vi "HBcenterFinder2Fids.vi"(0 "Operation":enum16{"Manual", "Automatic"}(ring)=enum."Automatic", 1 "Zone":enum16{"ZoneA", "ZoneB", "ZoneC", "ZoneD"}(ring), 2 "Autofocus":T3={"Enable"=TRUE, "InitialStepSize"=0.05, "Tolerance"=0.02, "Abort"=FALSE} {"Tolerance" format="%#_13g"}, 5 "Component":enum16{"BP", "Si", "HB", "HBonBP", "Other"}(ring)=enum."HB", 9 "VisibilityInCamera":enum16{"JoyStick", "AllVisible"}(ring)=enum."AllVisible", 11 "error in (no error)":errorcluster, 12 "Position":enum16{"1", "2"}(ring), 13 "SaveImagesLog":bool=TRUE) -> (4 "Output XYZU":string, 6 "Image":T4(plugin-control), 8 "Image 2":T4[](array[plugin-control]) caption="AllImages", 15 "error out":errorcluster)   [LabVIEW 2021]
uses:
  <vilib>/userDefined/High Color/IMAQdx.ctl
  <vilib>/Analysis/coordinate.llb/2D Cartesian Coordinate Rotation (Scalar).vi
  <vilib>/Analysis/baseanly.llb/Mean (DBL).vi
  include/GlobalVariables.vi
  <vilib>/Analysis/NI_AALPro.lvlib
  <vilib>/Analysis/NI_AALBase.lvlib
  <vilib>/vision/driver/NI_Vision_Acquisition_Software.lvlib
panel:
  out "JoyStickStatus":bool
  in  "YoffsetMidFid":dbl=3.5005
  in  "XoffsetMidFid":dbl
  out "DistFids":dbl=50.0
  out "AllMatches":T1(array[cluster]) {"Bounding Box"."y" format="%.2f"; "Bounding Box"."x" format="%.2f"; "Score" format="%.2f"; "Scale" format="%.2f"; "Angle" format="%.2f"; "Position"."y" format="%.2f"; "Position"."x" format="%.2f"}
  in  "Camera":T2="cam1"
  out "OutputFile":string
  out "spreadsheet string 2":string
  out "spreadsheet string":string
  in  "ModuleName":string="T1"
  out "SyringeY":dbl format="%#_7g"
  out "SyringeX":dbl format="%#_7g"
  in  "CamToSyringeYoffset":dbl=126.651
  in  "CamToSyringeXoffset":dbl=167.702
  out "FileUsedForFiducials":string
  out "UsedCoordinates":string
  out "CameraGcode":string
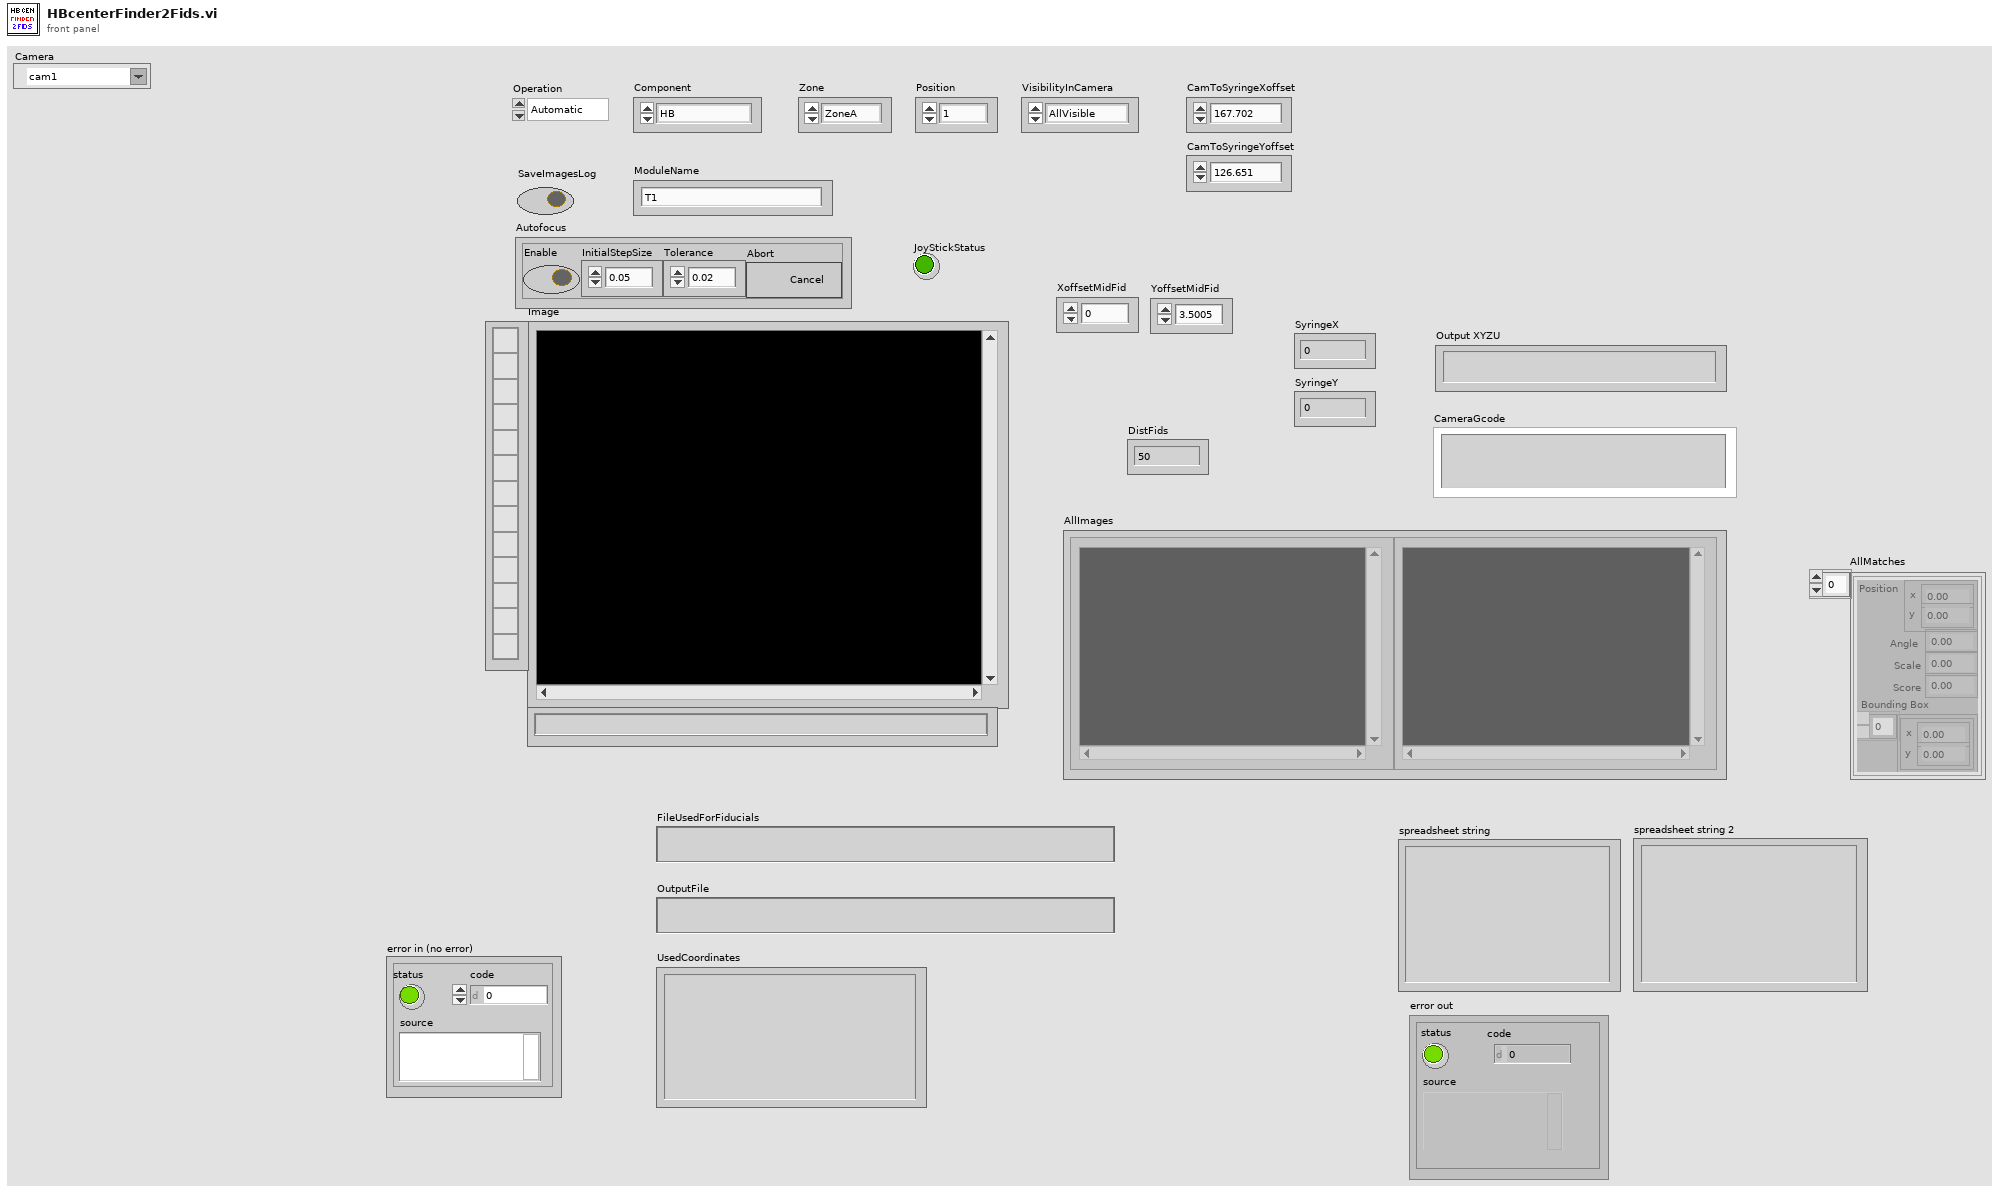
[diagram p1: front panel]
types:
  T1 = cluster{"Position":cluster{"x":sgl, "y":sgl}, "Angle":sgl, "Scale":sgl, "Score":sgl, "Bounding Box":cluster{"x":sgl, "y":sgl}[]}[]
  T2 = typedef "IMAQdx.ctl" = refnum<k21>
  T3 = cluster{"Enable":bool, "InitialStepSize":dbl, "Tolerance":dbl, "Abort":bool}
  T4 = typedef "IMAQ Image.ctl" = refnum<image>
  T5 = cluster{"Number of Matches Requested":i32, "Minimum Match Score":sgl, "Angle Ranges":cluster{"Start Angle":sgl, "End Angle":sgl}[]}
  T6 = typedef "Image Type" = u32
  T7 = typedef "IMAQ Circle" = cluster{"Center X":i32, "Center Y":i32, "Inner Radius":i32, "Outer Radius":i32, "Start Angle":dbl, "End Angle":dbl}
  T8 = enum16{"Left Button", "Center Button", "Right Button", "Window Close"}
  T9 = enum16{"open", "replace", "create", "open or create", "replace or create", "replace or create with confirmation"}
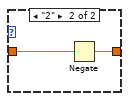
[diagram p2: hidden frame]
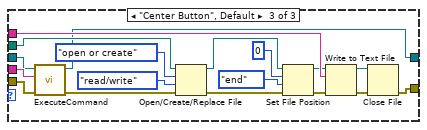
[diagram p5: hidden frame]
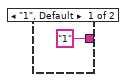
[diagram p6: hidden frame]
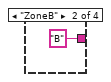
[diagram p7: hidden frame]
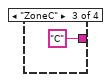
[diagram p8: hidden frame]
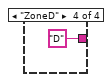
[diagram p9: hidden frame]
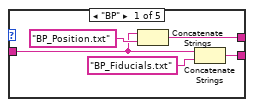
[diagram p10: hidden frame]
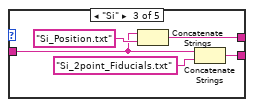
[diagram p11: hidden frame]
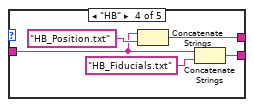
[diagram p12: hidden frame]
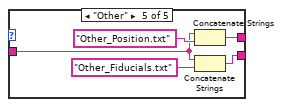
[diagram p13: hidden frame]
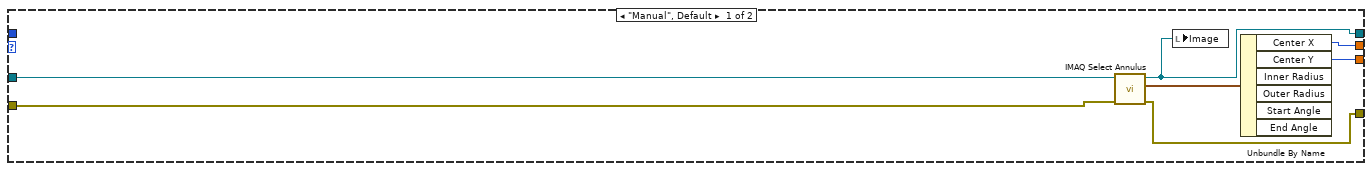
[diagram p14: hidden frame]
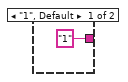
[diagram p16: hidden frame]
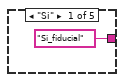
[diagram p17: hidden frame]
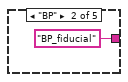
[diagram p18: hidden frame]
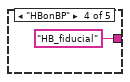
[diagram p19: hidden frame]
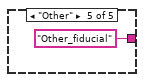
[diagram p20: hidden frame]
diagram:
  w49 = "%f" ("format string")
  w87 = "\t"
  w84 = i16 6 ("width (-)")
  # "Write the XYZU of the baseplate to a text file & move the gantry?"
  # "Prepare to move the gantry to see the center of baseplate in camera."
  # "AllVisble: Assumes that you know the coordinates of all corners (fiducials) well. No need for any adjustments.\nJoyStick: Use joystick at each point to make good image.\nClickMove: Use \"AdjustCamera\" panel and move the gantry stepwise. Click \"Done\" when you're satisfied with the picture."
  n1 = flat-sequence {
    tunnel: [w96] -> w45
    tunnel: w45 -> [w112]
    tunnel: [w111] -> w44
    tunnel: [w110] -> w42
    tunnel: [w109] -> w39
    tunnel: w44 -> [w164]
    tunnel: [w164] -> w43
    tunnel: w42 -> [w157]
    tunnel: [w152] -> w41
    tunnel: [w163] -> w40
    tunnel: w39 -> [w162]
    tunnel: [w162] -> w38
    tunnel: [w156] -> w30
    tunnel: [w155] -> w29
    tunnel: 2 -> [w191]
    tunnel: "VisibilityInCamera" -> [w184]
    tunnel: w43 -> [w182]
    tunnel: w41 -> [w174]
    tunnel: w40 -> [w181]
    tunnel: w38 -> [w180]
    tunnel: w30 -> [w172]
    tunnel: w29 -> [w173]
    tunnel: [w190] -> w28
    tunnel: [w189] -> w27
    tunnel: [w188] -> w26
    tunnel: [w187] -> w25
    tunnel: [w186] -> w24
    tunnel: [w185] -> w23
    tunnel: [w183] -> w22
    tunnel: [w180] -> w21
    tunnel: [w179] -> w20
    tunnel: [w171] -> w19
    tunnel: [w452] -> w36
    tunnel: [w453] -> w37
    tunnel: [w454] -> w54
    tunnel: [w455] -> w15
    tunnel: [w449] -> w16
    tunnel: [w456] -> _
    tunnel: [w457] -> w91
    tunnel: [w458] -> w50
    tunnel: [w459] -> w51
    tunnel: w28 -> [w459]
    tunnel: w27 -> [w458]
    tunnel: w26 -> [w457]
    tunnel: w25 -> [w456]
    tunnel: w24 -> [w450]
    tunnel: w23 -> [w455]
    tunnel: w22 -> [w454]
    tunnel: w21 -> [w453]
    tunnel: w20 -> [w452]
    tunnel: w19 -> [w451]
    frame #0 {
      n2 = case shown="\"ZoneA\", Default" "Zone" {
        tunnel: ["A" "B" "C" "D"] -> w100
        frame "ZoneA", Default {
        }
        frame "ZoneB" {
        }
        frame "ZoneC" {
        }
        frame "ZoneD" {
        }
      }
      n3 = case shown="\"2\"" "Position" {
        tunnel: ["1" "2"] -> w101
        frame "1", Default {
        }
        frame "2" {
        }
      }
      n4 = Concatenate Strings(w100, w101, "_" ("string")) -> (w96:string)
      "UsedCoordinates" <- ""
    }
    frame #1 {
      n5 = Concatenate Strings("C:\\Users\\TTUHEP\\Documents\\LabVIEW\\GantryPrograms\\", "Configs\\" ("string"), w112) -> (w119:string)
      n6 = case shown="\"HBonBP\"" "Component" {
        tunnel: w119 -> [w127 w132 w138 w143 w148]
        tunnel: [w128 w133 w140 w145 w150] -> w122
        tunnel: [w129 w134 w137 w142 w147] -> w109
        frame "BP" {
          n7 = Concatenate Strings(w127, "BP_Position.txt") -> (w129:string)
          n8 = Concatenate Strings(w127, "BP_Fiducials.txt") -> (w128:string)
        }
        frame "HBonBP" {
          n9 = Concatenate Strings(w132, "BP_Position.txt") -> (w134:string)
          n10 = Concatenate Strings(w132, "HBonBP_Fiducials.txt") -> (w133:string)
        }
        frame "Si" {
          n11 = Concatenate Strings(w138, "Si_Position.txt") -> (w137:string)
          n12 = Concatenate Strings(w138, "Si_2point_Fiducials.txt") -> (w140:string)
        }
        frame "HB" {
          n13 = Concatenate Strings(w143, "HB_Position.txt") -> (w142:string)
          n14 = Concatenate Strings(w143, "HB_Fiducials.txt") -> (w145:string)
        }
        frame "Other" {
          n15 = Concatenate Strings(w148, "Other_Position.txt") -> (w147:string)
          n16 = Concatenate Strings(w148, "Other_Fiducials.txt") -> (w150:string)
        }
      }
      "FileUsedForFiducials" <- w122
      "OutputFile" <- w109
      n17 = String To Path(string=w122) -> (path=w120:path)
      n18 = Concatenate Strings("This file does not exist:" ("ErrorMessage"), w122) -> (w123:string)
      n19 = call <vilib>:"Check if File or Folder Exists.vi"("error in (no error)"="error in (no error)", "path"=w120) -> ("error out"=w121:errorcluster, "file or folder exists?"=w124:bool, "dup path"=w111:path)  [unwired: 7 in]
      n20 = Not(x=w124) -> (.not. x?=w125:bool)
      n21 = call "AddError.vi"("NoErrorMessage"="InFile OK", "ErrorMessage"=w123, "error in"=w121, "code"=-995, "Error?"=w125) -> ("Error out"=w110:errorcluster)  [unwired: 6 in]
    }
    frame #2 {
      w158 = T6 0 items=["Grayscale (U8)", "Grayscale (I16)", "Grayscale (SGL)", "Complex (CSG)", "RGB (U32)", "HSL (U32)", "RGB (U64)", "Grayscale (U16)"] ("Image Type")
      # "Set the size of the window while selecting the point."
      n22 = call "IMAQ WindSize"("Scrollbars? (N)"=TRUE, "Width & Height"=cluster{"Width":i32, "Height":i32} {"Width"=1333, "Height"=1000}, "Window Number"=0) -> ()  [unwired: 3 in, 3 out]
      n23 = call "IMAQ Create"("Image Name"="name1" ("ImageName"), "Image Type"=w158, "error in (no error)"=w157) -> ("New Image"=w155:T4, "error out"=w160:errorcluster)  [unwired: 2 in]
      n24 = call "Connect.vi"("error in (no error)"=w157) -> ("error out"=w166:errorcluster, "controller"=w167:refnum<k24>)  [unwired: 9 in]
      n25 = call "ExecuteCommand.vi"("error in (no error)"=w166, "Command Code"="G90\nG1 Z0 F100", "controller in"=w167) -> ("error out"=w154:errorcluster, "controller out"=w163:refnum<k24>)  [unwired: 6 in, 1 out]
      n26 = call <vilib>:"IMAQdx Open Camera.vi"("error in"=w160, "Session In"="Camera") -> ("error out"=w153:errorcluster, "Session Out"=w156:T2)  [unwired: 8 in]
      n27 = Merge Errors(w154, w153) -> (w152:errorcluster)
    }
    frame #3 {
      n28 = local read "Autofocus"() -> (w176:T3)
      n29 = local read "Autofocus"() -> (w178:T3)
      n30 = Unbundle By Name(w178) -> ("Enable"=w177:bool)
      n31 = Unbundle By Name(w176) -> ("Abort"=w175:bool)
      n32 = for {
        N: w191 -> [_]
        tunnel: w181 -> [w252]
        tunnel: w182 -> [w235]
        tunnel: [w233] -> w190 mode=indexing
        tunnel: [w232] -> w189 mode=indexing
        tunnel: [w231] -> w188 mode=indexing
        tunnel: [w227] -> w187 mode=indexing
        tunnel: [w226] -> w185
        tunnel: w184 -> [w225]
        tunnel: w175 -> [w224]
        tunnel: w177 -> [w223]
        tunnel: [w219] -> w183
        tunnel: [w214] -> w179 mode=indexing
        shift-right: [w217] -> w186
        shift-left: w174 -> [w201]
        tunnel: w173 -> [w200]
        shift-right: [w194] -> w171
        shift-left: w172 -> [w193]
        i -> [w212]
        w203 = T6 6 items=["Grayscale (U8)", "Grayscale (I16)", "Grayscale (SGL)", "Complex (CSG)", "RGB (U32)", "HSL (U32)", "RGB (U64)", "Grayscale (U16)"] ("Image Type")
        # "Array of XY cluser"
        # "Z array"
        # "Y array"
        # "X array"
        # "Read text file line by line. Each line contains X,Y,Z coordinates for the gantry."
        n33 = call "GetArrayFmTxtFile.vi"("error in"=w201, "LineNo."=w212, "TextFile"=w235) -> ("error out"=w234:errorcluster, "Array"=w259:dbl[])
        n34 = Index Array(array=w259, index=0) -> (element=w254:dbl)
        n35 = Index Array(array=w259, index=1) -> (element=w253:dbl)
        n36 = Index Array(array=w259, index=2) -> (element=w255:dbl)
        n37 = call "Move.vi"("X"=w254, "Absolute"=TRUE, "Y"=w253, "Z"=w255, "SpeedXY (mm/s)"=100.0, "SpeedZ (mm/s)"=100.0, "Move Z first"=FALSE) -> ("Position Gcode"=w251:string)  [unwired: 8 in]
        n38 = call "ExecuteCommand.vi"("error in (no error)"=w234, "Command Code"=w251, "controller in"=w252) -> ("error out"=w199:errorcluster, "controller out"=w250:refnum<k24>)  [unwired: 6 in, 1 out]
        n39 = call <vilib>:"IMAQdx Snap2.vi"("error in"=w199, "Image In"=w200, "Session In"=w193) -> ("error out"=w198:errorcluster, "Image Out"=w196:T4, "Session Out"=w197:T2)  [unwired: 6 in]
        n40 = local write "Image"(w196) -> ()
        n41 = case shown="\"JoyStick\", Default" w225 {
          tunnel: w197 -> [w367 w418]
          tunnel: w250 -> [w384 w430]
          tunnel: w198 -> [w382 w431]
          tunnel: [w363 w419] -> w221
          tunnel: [w371 w425] -> w239
          tunnel: [w372 w423] -> w195
          tunnel: w224 -> [w375 w428]
          tunnel: w223 -> [w369 w429]
          tunnel: "name1" ("ImageName") -> [w368 w417]
          tunnel: w196 -> [w366 w416]
          tunnel: [w362 w415] -> w194
          frame "JoyStick", Default {
            # "Use joystick to go to a position where camera sees good image."
            n42 = while {
              tunnel: [w407] -> w364
              tunnel: w384 -> [w414]
              tunnel: [w412] -> w380
              tunnel: [w414] -> w381
              tunnel: w382 -> [w413]
              tunnel: w367 -> [w411]
              tunnel: w366 -> [w410]
              tunnel: [w409] -> w365
              stop <- w408 continue-if-true
              n43 = call <vilib>:"IMAQdx Snap2.vi"("error in"=w413, "Image In"=w410, "Session In"=w411) -> ("error out"=w412:errorcluster, "Image Out"=w407:T4, "Session Out"=w409:T2)  [unwired: 6 in]
              n44 = local write "Image"(w407) -> ()
              n45 = global write "GlobalVariables.vi" "Image"(w407) -> ()
              n46 = local read "JoyStickStatus"() -> (w408:bool)
            }
            n47 = call "ExecuteCommand.vi"("error in (no error)"=w382, "Command Code"="JOYSTICK 2D RESET\nJOYSTICK 2D AXISGROUP 1 Y X\nJOYSTICK 2D AXISGROUP 2 Y Z\nJOYSTICK 2D ON", "controller in"=w384) -> ("error out"=w383:errorcluster, "controller out"=w360:refnum<k24>)  [unwired: 6 in, 1 out]
            n48 = call <vilib>:"Clear Errors.vi"("error in (no error)"=w383) -> ()  [unwired: 5 in, 2 out]
            n49 = call "GetGantryPosition.vi"("error in (no error)"=w380, "Controller In"=w381) -> ("error out"=w376:errorcluster, "controller out"=w374:refnum<k24>, "Position_XYZ"=w370:string)  [unwired: 3 in, 4 out]
            n50 = Not A Number/Path/Refnum?(number/path/refnum=w360) -> (NaN/Path/Refnum?=w361:bool)
            n51 = case shown="False" w369 {
              tunnel: w376 -> [w390 w406]
              tunnel: w375 -> [_ w399]
              tunnel: w374 -> [w388 w400]
              tunnel: [w389 w404] -> w373
              tunnel: [w390 w403] -> w372
              tunnel: [w388 w402] -> w371
              tunnel: w370 -> [w389 _]
              tunnel: w368 -> [_ _]
              tunnel: w365 -> [w386 w394]
              tunnel: w364 -> [w387 w393]
              tunnel: [w387 w392] -> w363
              tunnel: [w386 w391] -> w362
              frame False {
              }
              frame True {
                n52 = local read "Autofocus"() -> (w397:T3)
                n53 = Unbundle By Name(w397) -> ("InitialStepSize"=w395:dbl, "Tolerance"=w396:dbl)
                n54 = call "Autofocus.vi"("controller in"=w400, "AbortAutoFocus"=w399, "ImageIn"=w393, "SafeMaxZ"=80.0, "InitialStepSize"=w395, "Tolerance"=w396, "error in (no error)"=w406, "SessionIn"=w394) -> ("controller out"=w405:refnum<k24>, "Image"=w392:T4, "Session Out"=w391:T2, "error out"=w401:errorcluster)  [unwired: 2 in, 2 out]
                n55 = local write "Image"(w392) -> ()
                n56 = call "GetGantryPosition.vi"("error in (no error)"=w401, "Controller In"=w405) -> ("error out"=w403:errorcluster, "controller out"=w402:refnum<k24>, "Position_XYZ"=w404:string)  [unwired: 3 in, 4 out]
              }
            }
            n57 = local write "JoyStickStatus"(w361) -> ()
            n58 = local read "UsedCoordinates"() -> (w378:string)
            n59 = Concatenate Strings(w378, "\r", w373) -> (w379:string)
            n60 = local write "UsedCoordinates"(w379) -> ()
          }
          frame "AllVisible" {
            # "No need to move gantry to take a good pic."
            n61 = case shown="False" w429 {
              tunnel: w428 -> [_ w443]
              tunnel: [w435 w446] -> w424
              tunnel: [w434 w448] -> w426
              tunnel: w431 -> [w435 w447]
              tunnel: w430 -> [w434 w445]
              tunnel: [w433 w442] -> w419
              tunnel: w418 -> [w432 w438]
              tunnel: w417 -> [_ _]
              tunnel: w416 -> [w433 w437]
              tunnel: [w432 w436] -> w415
              frame False {
              }
              frame True {
                n62 = local read "Autofocus"() -> (w441:T3)
                n63 = Unbundle By Name(w441) -> ("InitialStepSize"=w440:dbl, "Tolerance"=w439:dbl)
                n64 = call "Autofocus.vi"("controller in"=w445, "AbortAutoFocus"=w443, "ImageIn"=w437, "SafeMaxZ"=80.0, "InitialStepSize"=w440, "Tolerance"=w439, "error in (no error)"=w447, "SessionIn"=w438) -> ("controller out"=w448:refnum<k24>, "Image"=w442:T4, "Session Out"=w436:T2, "error out"=w446:errorcluster)  [unwired: 2 in, 2 out]
                n65 = local write "Image"(w442) -> ()
              }
            }
            n66 = local read "UsedCoordinates"() -> (w421:string)
            n67 = call "GetGantryPosition.vi"("error in (no error)"=w424, "Controller In"=w426) -> ("error out"=w423:errorcluster, "controller out"=w425:refnum<k24>, "Position_XYZ"=w422:string)  [unwired: 3 in, 4 out]
            n68 = Concatenate Strings(w421, "\r", w422) -> (w420:string)
            n69 = local write "UsedCoordinates"(w420) -> ()
          }
        }
        n70 = case shown="\"Automatic\"" "Operation" {
          tunnel: [w267 w278] -> w247
          tunnel: [w266 w277] -> w246
          tunnel: [w268 w286] -> w245
          tunnel: w195 -> [w263 w302]
          tunnel: w221 -> [w265 w307]
          tunnel: w212 -> [_ _]
          tunnel: [w264 w284] -> w213
          frame "Manual", Default {
            n71 = call "IMAQ Select Annulus"("error in (no error)"=w263, "Image In"=w265) -> ("error out"=w268:errorcluster, "Annulus"=w269:T7, "Image Out (duplicate)"=w264:T4)  [unwired: 6 in, 1 out]
            n72 = local write "Image"(w264) -> ()
            n73 = Unbundle By Name(w269) -> ("Center X"=w267:i32, "Center Y"=w266:i32)  [unwired: 4 out]
          }
          frame "Automatic" {
            w282 = sgl 50.0 ("y")
            w300 = ""
            n74 = local read "Position"() -> (w289:enum16{"1", "2"})
            n75 = case shown="\"2\"" w289 {
              tunnel: ["1" "2"] -> w288
              frame "1", Default {
              }
              frame "2" {
              }
            }
            n76 = local read "Component"() -> (w304:enum16{"BP", "Si", "HB", "HBonBP", "Other"})
            n77 = case shown="\"HB\"" w304 {
              tunnel: ["Si_fiducial" "BP_fiducial" "HB_fiducial" "HB_fiducial" "Other_fiducial"] -> w303
              tunnel: w288 -> [_ _ _ _ _]
              frame "Si" {
              }
              frame "BP" {
              }
              frame "HB" {
              }
              frame "HBonBP" {
              }
              frame "Other" {
              }
            }
            n78 = Concatenate Strings("Could not parse/find this template file for pattern recognition:" ("ErrorMessage"), w303) -> (w295:string)
            n79 = call "JSONfileReader.vi"("error in"=w302, "Variant"=w300, "ItemName"=w303, "FileIn"=path "C:/Users/TTUHEP/Documents/LabVIEW/GantryPrograms/Configs/PatternRecognTemplateMaps.json" ("PatterRecognTemplateMap")) -> ("error out"=w292:errorcluster, "Data"=w301:variant, "Found"=w298:bool)
            n80 = Not(x=w298) -> (.not. x?=w297:bool)
            n81 = Variant To Data(error in=w292, type=w300, Variant=w301) -> (data=w299:string, error out=w291:errorcluster)
            n82 = call "AddError.vi"("NoErrorMessage"="Template file name found from json.", "ErrorMessage"=w295, "error in"=w291, "code"=-902, "Error?"=w297) -> ("Error out"=w290:errorcluster)  [unwired: 6 in]
            n83 = call "PatternRecognition.vi"("error in (no error)"=w290, "MatchParameters"=T5 {"Number of Matches Requested"=1, "Minimum Match Score"=500.0, "Angle Ranges"=[{"Start Angle"=0.0, "End Angle"=0.0}]}, "ImageIn"=w307, "TemplateFileName"=w299) -> ("error out"=w273:errorcluster, "AllMatches"=→"AllMatches":T1, "Position"=w306:cluster{"x":sgl, "y":sgl}, "ImageFoundPattern"=w285:T4, "Number of Matches"=w287:i32)  [unwired: 2 in]
            n84 = Equal To 0?(x=w287) -> (x = 0?=w283:bool)
            n85 = Unbundle(w306) -> ("x"=w276:sgl, "y"=w275:sgl)
            n86 = call <vilib>:"Clear Errors.vi"("error in (no error)"=w273, "specific error code to clear (0: all)"=-903) -> ("error out"=w272:errorcluster)  [unwired: 4 in, 1 out]
            n87 = Less?(x=w276, y=w282) -> (x < y?=w281:bool)
            n88 = Less?(x=w275, y=w282) -> (x < y?=w280:bool)
            n89 = Compound Arithmetic op=OR(w283, w281, w280) -> (w279:bool)
            n90 = case shown="True" w279 {
              tunnel: w272 -> [w311 w318]
              tunnel: [w311 w317] -> w286
              tunnel: w285 -> [w310 w316]
              tunnel: [w310 w315] -> w284
              tunnel: [w309 w313] -> w278
              tunnel: [w308 w312] -> w277
              tunnel: w276 -> [w309 _]
              tunnel: w275 -> [w308 _]
              frame False {
              }
              frame True {
                n91 = call "IMAQ Select Annulus"("Window Number (0...15)"=0, "error in (no error)"=w318, "Image In"=w316) -> ("error out"=w317:errorcluster, "Annulus"=w314:T7, "Image Out (duplicate)"=w315:T4)  [unwired: 5 in, 1 out]
                n92 = Unbundle(w314) -> ("Center X"=w313:i32, "Center Y"=w312:i32)  [unwired: 4 out]
              }
            }
          }
        }
        n93 = Number To Decimal String(number=w212) -> (decimal integer string=w211:string)  [unwired: 1 in]
        n94 = Concatenate Strings("imgTemp" ("string"), w211) -> (w208:string)
        n95 = call "GetPixelToGantryRelPosition.vi"("error in (no error)"=w245, "PixelY"=w246, "PixelX"=w247) -> ("error out"=w206:errorcluster, "YmmRelGH"=w243:dbl, "XmmRelGH"=w244:dbl)
        n96 = call "IMAQ Create"("Image Name"=w208, "Image Type"=w203, "error in (no error)"=w206) -> ("New Image"=w207:T4, "error out"=w205:errorcluster)  [unwired: 2 in]
        n97 = call "IMAQ Copy"("error in (no error)"=w205, "Image Dst"=w207, "Image Src"=w213) -> ("error out"=w204:errorcluster, "Image Dst Out"=w209:T4)  [unwired: 3 in]
        n98 = Build Array(w209) -> (w214:T4[])
        n99 = flat-sequence {
          tunnel: w204 -> [w351]
          tunnel: [w351] -> w249
          tunnel: w239 -> [w350]
          tunnel: [w350] -> w248
          tunnel: [w359] -> w218
          tunnel: [w358] -> w242
          tunnel: [w357] -> w241
          tunnel: [w356] -> w226
          tunnel: [w355] -> w240
          tunnel: w249 -> [w354]
          tunnel: w248 -> [w353]
          frame #0 {
            n100 = Wait (ms)(milliseconds to wait=u32 1000) -> ()  [unwired: 1 out]
          }
          frame #1 {
            n101 = call "GetGantryPosition.vi"("error in (no error)"=w354, "Controller In"=w353) -> ("error out"=w359:errorcluster, "Position Y"=w358:dbl, "Position X"=w357:dbl, "controller out"=w356:refnum<k24>, "Position Z"=w355:dbl)  [unwired: 3 in, 2 out]
          }
        }
        n102 = Add(x=w244, y=w241) -> (x+y=w238:dbl)
        n103 = Add(x=w243, y=w242) -> (x+y=w237:dbl)
        n104 = case shown="True" "SaveImagesLog" {
          tunnel: w213 -> [w327 w345]
          tunnel: w212 -> [_ w343]
          tunnel: ["" w335] -> w219
          tunnel: w218 -> [w328 w334]
          tunnel: [w328 w333] -> w217
          tunnel: [w327 w332] -> w202
          frame False {
          }
          frame True {
            w337 = "C:\\Users\\TTUHEP\\Documents\\LabVIEW\\GantryPrograms\\LogFiles\\CalibrationData\\"
            n105 = local read "Component"() -> (w331:enum16{"BP", "Si", "HB", "HBonBP", "Other"})
            n106 = case shown="\"HB\"" w331 {
              tunnel: ["BP_fiducial" "Si_fiducial" "Other_fiducial" "HB_fiducial"] -> w330
              frame "BP" {
              }
              frame "Si", Default {
              }
              frame "Other" {
              }
              frame "HB" {
              }
            }
            n107 = Number To Decimal String(number=w343) -> (decimal integer string=w341:string)  [unwired: 1 in]
            n108 = Concatenate Strings(w337, "ModuleName") -> (w335:string)
            n109 = Concatenate Strings(w337, "ModuleName", w330, "Image" ("string"), w341, ".png" ("string")) -> (w339:string)
            n110 = String To Path(string=w339) -> (path=w338:path)
            n111 = call-poly "IMAQ Write File 2"("error in (no error)"=w334, "Image Quality"=u32 1000, "File Path"=w338, "Image"=w345) -> ("error out"=w333:errorcluster, "Image Out (duplicate)"=w332:T4)  [unwired: 6 in]
          }
        }
        "Image" <- w202
        n112 = call-poly <vilib>:"2D Cartesian Coordinate Rotation.vi"("theta"=0.0, "y"=w237, "x"=w238) -> ("y out"=w229:dbl, "x out"=w230:dbl)  [unwired: 6 in, 1 out]
        n113 = global write "GlobalVariables.vi" "Image"(w202) -> ()
        n114 = Bundle("x out"=w230, "y out"=w229) -> (w228:cluster{"x out":dbl, "y out":dbl})  [unwired: 1 in]
        n115 = Build Array(w228) -> (w227:cluster{"x out":dbl, "y out":dbl}[])
        n116 = Build Array(w229) -> (w232:dbl[])
        n117 = Build Array(w230) -> (w233:dbl[])
        n118 = Build Array(w240) -> (w231:dbl[])
        "JoyStickStatus" <- TRUE ("NaN/Path/Refnum?")
      }
    }
    frame #4 {
      n119 = call <vilib>:"IMAQdx Close Camera.vi"("error in"=w450, "Session In"=w451) -> ("error out"=w449:errorcluster)  [unwired: 9 in]
    }
  }
  n120 = Array To Spreadsheet String(array=w50, 3:w49) -> (spreadsheet string=→"spreadsheet string 2":string)  [unwired: 1 in]
  n121 = Array To Spreadsheet String(array=w51, 3:w49) -> (spreadsheet string=→"spreadsheet string":string)  [unwired: 1 in]
  n122 = String To Path(string=w37) -> (path=w46:path)
  n123 = Index Array(array=w36, index (col)=0 ("disabled index (col)")) -> (element=→"Image 2":T4[])  [unwired: 1 in]
  n124 = Index Array "Y"(array=w50, index (col)=0 ("disabled index (col)")) -> (element=w17:dbl[])  [unwired: 1 in]
  n125 = Index Array "X"(array=w51, index (col)=0 ("disabled index (col)")) -> (element=w18:dbl[])  [unwired: 1 in]
  n126 = Index Array "Z"(array=w91, index (col)=0 ("disabled index (col)")) -> (element=w90:dbl[])  [unwired: 1 in]
  n127 = formula code="float64 xMid = 0.5*(xin[0]+xin[1]);\nfloat64 yMid = 0.5*(yin[0]+yin[1]);\nfloat64 dist = sqrt((xin[0]-xin[1])*(xin[0]-xin[1]) + (yin[0]-yin[1])*(yin[0]-yin[1]));\nfloat64 angle = 90.0 - (asin(abs(yin[0] - yin[1])/dist)*180.0/3.14159);\nif((xin[0]-xin[1])/(yin[0]-yin[1]) <=0)\n  angle = angle;\nelse\n  angle = -angle;"("xin"=w18, "yin"=w17) -> ("xMid"=w11:dbl, "yMid"=w7:dbl, "angle"=w4:dbl, "dist"=→"DistFids":dbl)
  n128 = local read "Position"() -> (w3:enum16{"1", "2"})
  n129 = case shown="\"1\", Default" w3 {
    tunnel: "YoffsetMidFid" -> [w460 w462]
    tunnel: [w460 w461] -> w1
    frame "1", Default {
    }
    frame "2" {
      n130 = Negate(x=w462) -> (-x=w461:dbl)
    }
  }
  n131 = Negate(x=w4) -> (-x=w5:dbl)
  n132 = call-poly <vilib>:"Mean.vi"("X"=w90) -> ("mean"=w67:dbl)  [unwired: 1 out]
  n133 = expression code="(x/180.0)*pi" "degrees to radians"(w5) -> (w12:dbl)
  n134 = call-poly <vilib>:"2D Cartesian Coordinate Rotation.vi"("theta"=w12, "y"=w1, "x"="XoffsetMidFid") -> ("y out"=w8:dbl, "x out"=w10:dbl)  [unwired: 6 in, 1 out]
  n135 = Add(x=w11, y=w10) -> (x+y=w9:dbl)
  n136 = Add(x=w7, y=w8) -> (x+y=w6:dbl)
  n137 = Number To Fractional String(number=w9, precision (6)=w84) -> (F-format string=w89:string)  [unwired: 2 in]
  n138 = Number To Fractional String(number=w6, precision (6)=w84) -> (F-format string=w88:string)  [unwired: 2 in]
  n139 = Number To Fractional String(number=w67, precision (6)=w84) -> (F-format string=w83:string)  [unwired: 2 in]
  n140 = call "CameraXYusingGantryHeadXY.vi"("GantryY"=w6, "GantryX"=w9) -> ("CamY"=w60:dbl, "CamX"=w62:dbl)
  n141 = Number To Fractional String(number=w4, precision (6)=i16 4 ("width (-)")) -> (F-format string=w85:string)  [unwired: 2 in]
  n142 = call "Move.vi"("X"=w62, "Absolute"=TRUE, "Y"=w60, "Z"=w67, "SpeedXY (mm/s)"=100.0, "SpeedZ (mm/s)"=50.0, "Move Z first"=TRUE) -> ("Position Gcode"=w70:string)  [unwired: 8 in]
  "CameraGcode" <- w70
  n143 = Add(x="CamToSyringeYoffset", y=w60) -> (x+y=→"SyringeY":dbl)
  n144 = Concatenate Strings(w89, w87, w88, w87, w83, w87, w85, "\r") -> (w81:string)
  "Output XYZU" <- w81
  n145 = Add(x="CamToSyringeXoffset", y=w62) -> (x+y=→"SyringeX":dbl)
  n146 = Concatenate Strings("Overwrite/Append ", w81, " to file ", w37, " ?" ("string")) -> (w78:string)
  n147 = call <vilib>:"Three Button Dialog.vi"("Right Button Text (\"Cancel\")"="Do nothing" ("Right Button Text (\"Cancel\")"), "Center Button Text (\"No\")"="Append" ("Center Button Text (\"No\")"), "Left Button Text (\"Yes\")"="Overwrite" ("Left Button Text (\"Yes\")"), "message"=w78) -> ("Which Button?"=w77:T8)  [unwired: 7 in]
  n148 = case shown="\"Left Button\"" w77 {
    tunnel: w81 -> [w470 _ w492]
    tunnel: w46 -> [w469 _ w491]
    tunnel: w16 -> [w468 w478 w490]
    tunnel: w70 -> [w467 _ w489]
    tunnel: w15 -> [w466 w477 w488]
    tunnel: [w463 w478 w479] -> w56
    tunnel: [w465 w477 w487] -> w69
    frame "Left Button" {
      n149 = call "ExecuteCommand.vi"("error in (no error)"=w468, "Command Code"=w467, "controller in"=w466) -> ("error out"=w464:errorcluster, "controller out"=w465:refnum<k24>)  [unwired: 6 in, 1 out]
      n150 = Open/Create/Replace File(file path (use dialog)=w469, error in=w464, operation (0:open)=T9."replace or create", access (0:read/write)=enum16{"read/write", "read-only", "write-only"}."read/write") -> (refnum out=w476:refnum<file>, error out=w473:errorcluster)  [unwired: 2 in, 1 out]
      n151 = Write to Text File(file (use dialog)=w476, text=w470, error in=w473) -> (refnum out=w471:refnum<file>, error out=w472:errorcluster)  [unwired: 1 in, 1 out]
      n152 = Close File(refnum=w471, error in=w472) -> (error out=w463:errorcluster)  [unwired: 1 out]
    }
    frame "Right Button" {
    }
    frame "Center Button", Default {
      n153 = call "ExecuteCommand.vi"("error in (no error)"=w490, "Command Code"=w489, "controller in"=w488) -> ("error out"=w480:errorcluster, "controller out"=w487:refnum<k24>)  [unwired: 6 in, 1 out]
      n154 = Open/Create/Replace File(file path (use dialog)=w491, error in=w480, operation (0:open)=T9."open or create", access (0:read/write)=enum16{"read/write", "read-only", "write-only"}."read/write") -> (refnum out=w484:refnum<file>, error out=w482:errorcluster)  [unwired: 2 in, 1 out]
      n155 = Set File Position(offset (in bytes) (0)=i64 0, refnum=w484, from (0:start)=enum16{"start", "end", "current"}."end", error in=w482) -> (refnum out=w483:refnum<file>, error out=w481:errorcluster)
      n156 = Write to Text File(file (use dialog)=w483, text=w492, error in=w481) -> (refnum out=w493:refnum<file>, error out=w494:errorcluster)  [unwired: 1 in, 1 out]
      n157 = Close File(refnum=w493, error in=w494) -> (error out=w479:errorcluster)  [unwired: 1 out]
    }
  }
  n158 = call "CaptureImage.vi"("Camera"=T2 "cam1", "ImageName"="CurrImage", "Draw50MicroCircleAtCenter"=TRUE, "error in (no error)"=w56) -> ("Image"=w33:T4, "error out"=w55:errorcluster)  [unwired: 3 in]
  n159 = local write "Image"(w33) -> ()
  n160 = global write "GlobalVariables.vi" "Image"(w33) -> ()
  n161 = call "Disconnect.vi"("error in (no error)"=w55, "controller"=w69) -> ("error out"=w52:errorcluster)  [unwired: 9 in]
  n162 = local read "SaveImagesLog"() -> (w57:bool)
  n163 = case shown="True" w57 {
    tunnel: w52 -> [w497 w512]
    tunnel: w54 -> [_ w505]
    tunnel: w33 -> [_ w500]
    tunnel: [w497 w498] -> w53
    frame False {
    }
    frame True {
      n164 = Concatenate Strings(w505, "UsedXYZ.txt") -> (w510:string)
      n165 = local read "UsedCoordinates"() -> (w507:string)
      n166 = Concatenate Strings(w505, "CenterImage.png") -> (w503:string)
      n167 = String To Path(string=w510) -> (path=w509:path)
      n168 = String To Path(string=w503) -> (path=w501:path)
      n169 = Open/Create/Replace File(file path (use dialog)=w509, error in=w512, operation (0:open)=T9."open or create", access (0:read/write)=enum16{"read/write", "read-only", "write-only"}."read/write") -> (refnum out=w508:refnum<file>, error out=w516:errorcluster)  [unwired: 2 in, 1 out]
      n170 = Write to Text File(file (use dialog)=w508, text=w507, error in=w516) -> (refnum out=w506:refnum<file>, error out=w515:errorcluster)  [unwired: 1 in, 1 out]
      n171 = Close File(refnum=w506, error in=w515) -> (error out=w499:errorcluster)  [unwired: 1 out]
      n172 = call-poly "IMAQ Write File 2"("error in (no error)"=w499, "Image Quality"=u32 1000, "File Path"=w501, "Image"=w500) -> ("error out"=w498:errorcluster)  [unwired: 6 in, 1 out]
    }
  }
  "error out" <- w53
